vi "Set the Address.vi"() -> ()   [LabVIEW 2018, in "Huber Unistat 410 TCU.lvlib"]
uses:
  Huber Unistat 410 TCU.lvlib
  Huber Unistat 410 RS485 Settings.ctl
  <vilib>/Instr/_visa.llb/VISA Configure Serial Port (Instr).vi
  <vilib>/regexp/Match Regular Expression.xnode
panel:
  in  "New Address":i8 min=0 max=99 format="%02.0f"
  out "Huber Unistat 410 Settings 2":T1 {"Address" min=0 max=99}
  in  "Huber Unistat 410 Settings":T1 {"Address" min=0 max=99}
  in  "Internal?":bool
  out "Connection Error":bool
  out "error out":errorcluster
  in  "error in (no error)":errorcluster
  out "read string":string
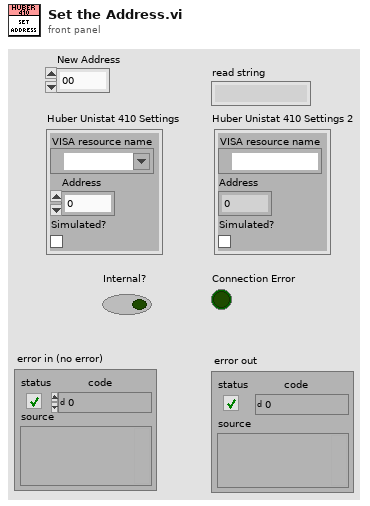
[diagram p1: front panel]
types:
  T1 = typedef "Huber Unistat 410 TCU.lvlib/Huber Unistat 410 RS485 Settings.ctl" = cluster{"VISA resource name":refnum<visa-resource-name>, "Address":i8, "Simulated?":bool}
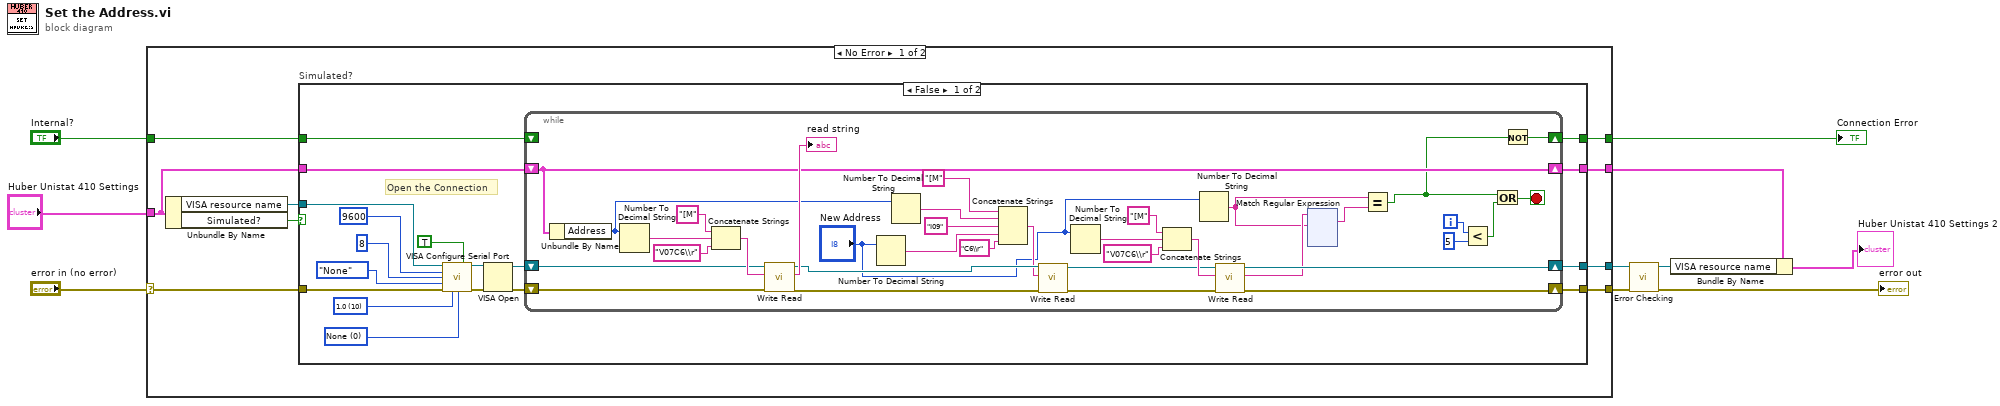
[diagram p0: block diagram]
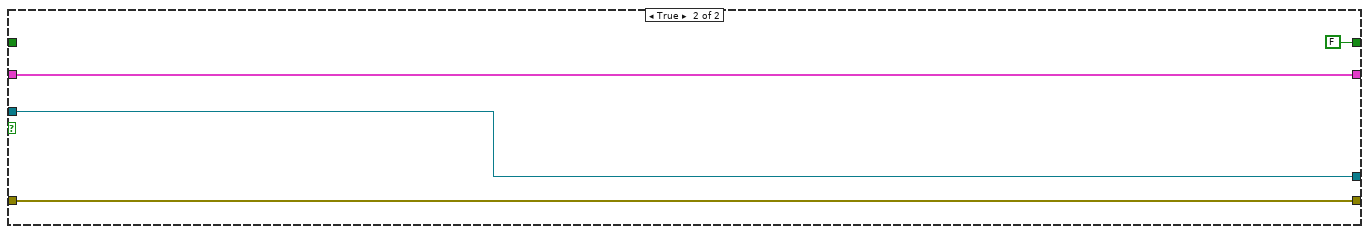
[diagram p2: hidden frame]
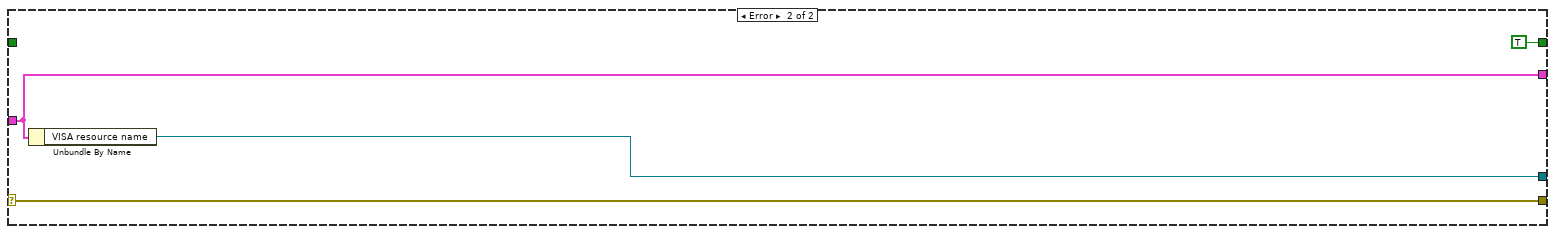
[diagram p3: hidden frame]
diagram:
  n1 = case shown="No Error" "error in (no error)" {
    selector: "error in (no error)" -> [w19 w194]
    tunnel: "Huber Unistat 410 Settings" -> [w13 w191]
    tunnel: [w18 w194] -> w8
    tunnel: [w16 w193] -> w9
    tunnel: [w14 TRUE] -> w5
    tunnel: [w12 w191] -> w4
    tunnel: "Internal?" -> [w11 _]
    frame No Error {
      n2 = Unbundle By Name(w13) -> ("VISA resource name"=w17:refnum<visa-resource-name>, "Simulated?"=w15:bool)
      n3 = case "Simulated?" shown="False" w15 {
        tunnel: w19 -> [w32 w190]
        tunnel: [w26 w190] -> w18
        tunnel: [w20 w189] -> w16
        tunnel: w17 -> [w31 w189]
        tunnel: [w28 FALSE] -> w14
        tunnel: w13 -> [w29 w187]
        tunnel: [w27 w187] -> w12
        tunnel: w11 -> [w25 _]
        frame False {
          w33 = u16 0 items=["None", "XON/XOFF", "RTS/CTS", "XON/XOFF & RTS/CTS", "DTR/DSR", "XON/XOFF & DTR/DSR"] ("flow control (0:none)")
          w34 = u16 10 items=["1.0"=10, "1.5"=15, "2.0"=20] ("stop bits (10: 1 bit)")
          # "Open the Connection"
          n4 = call-poly "VISA Configure Serial Port"("VISA resource name"=w31, "Enable Termination\nChar (T)"=TRUE ("Enable Termination\nChar (T)"), "baud rate (9600)"=u32 9600, "data bits (8)"=u16 8, "parity (0:none)"=enum16{"None", "Odd", "Even", "Mark", "Space"}."None", "error in (no error)"=w32, "stop bits (10: 1 bit)"=w34, "flow control (0:none)"=w33) -> ("VISA resource name out"=w23:refnum<visa-resource-name>, "error out"=w24:errorcluster)  [unwired: 6 in]
          n5 = VISA Open(error in (no error)=w24, VISA resource name=w23) -> (VISA resource name=w21:refnum<visa-resource-name>, error out=w22:errorcluster)  [unwired: 3 in]
          n6 = while {
            shift-right: [w44] -> w26
            shift-left: w22 -> [w66]
            shift-right: [w45] -> w20
            shift-left: w21 -> [w65]
            shift-right: [w56] -> w27
            shift-left: w29 -> [w56]
            shift-right: [w39] -> w28
            shift-left: w25 -> [_]
            i -> [w70]
            stop <- w67 stop-if-true
            n7 = Unbundle By Name(w56) -> ("Address"=w55:i8)
            n8 = Number To Decimal String(number=w55) -> (decimal integer string=w62:string)  [unwired: 1 in]
            n9 = Concatenate Strings("[M" ("string"), w62, "V07C6\\r" ("string")) -> (w72:string)
            n10 = call "Write Read.vi"("error in (no error)"=w66, "write string"=w72, "VISA Refnum in"=w65) -> ("error out"=w60:errorcluster, "read string"=→"read string":string, "VISA Refnum out"=w61:refnum<visa-resource-name>)  [unwired: 6 in]
            n11 = Number To Decimal String(number="New Address") -> (decimal integer string=w54:string)  [unwired: 1 in]
            n12 = Number To Decimal String(number=w55) -> (decimal integer string=w59:string)  [unwired: 1 in]
            n13 = Concatenate Strings("[M" ("string"), w59, "I09" ("string"), w54, "C6\\r" ("string")) -> (w52:string)
            n14 = call "Write Read.vi"("error in (no error)"=w60, "write string"=w52, "VISA Refnum in"=w61) -> ("error out"=w46:errorcluster, "VISA Refnum out"=w47:refnum<visa-resource-name>)  [unwired: 6 in, 1 out]
            n15 = Number To Decimal String(number="New Address") -> (decimal integer string=w48:string)  [unwired: 1 in]
            n16 = Concatenate Strings("[M" ("string"), w48, "V07C6\\r" ("string")) -> (w51:string)
            n17 = Number To Decimal String(number="New Address") -> (decimal integer string=w41:string)  [unwired: 1 in]
            n18 = call "Write Read.vi"("error in (no error)"=w46, "write string"=w51, "VISA Refnum in"=w47) -> ("error out"=w44:errorcluster, "read string"=w43:string, "VISA Refnum out"=w45:refnum<visa-resource-name>)  [unwired: 6 in]
            n19 = xnode "Match Regular Expression"("input string"=w43, "regular expression"=w41) -> ("whole match"=w40:string)  [unwired: 4 in, 4 out]
            n20 = Equal?(x=w41, y=w40) -> (x = y?=w38:bool)
            n21 = Less?(x=w70, y=5) -> (x < y?=w68:bool)
            n22 = Or(x=w38, y=w68) -> (x .or. y?=w67:bool)
            n23 = Not(x=w38) -> (.not. x?=w39:bool)
          }
        }
        frame True {
        }
      }
    }
    frame Error {
      n24 = Unbundle By Name(w191) -> ("VISA resource name"=w193:refnum<visa-resource-name>)
    }
  }
  "Connection Error" <- w5
  n25 = call "Error Checking.vi"("error in (no error)"=w8, "VISA resource name"=w9) -> ("error out"=→"error out":errorcluster, "VISA resource name"=w6:refnum<visa-resource-name>)  [unwired: 7 in, 1 out]
  n26 = Bundle By Name(cluster=w4, "VISA resource name"=w6) -> (→"Huber Unistat 410 Settings 2":T1)
